vi "Asylum_Driver_InitializeLithographyObject.vi"(6 "Z Setpoint":dbl format="%#_13g", 8 "error in (no error)":errorcluster, 9 "Offsets":cluster{"X":dbl, "Y":dbl}, 10 "Pattern Data":T2={"Name"="", "Litho"=[], "Set Resistance"=enum."1G ohm"}, 11 "Application":refnum<k7>) -> (0 "error out":errorcluster, 3 "Application":refnum<k7>)   [LabVIEW 2020]
uses:
  <userlib>/LevyLab/Relay Box/Type_defs/Resistor--enum.ctl
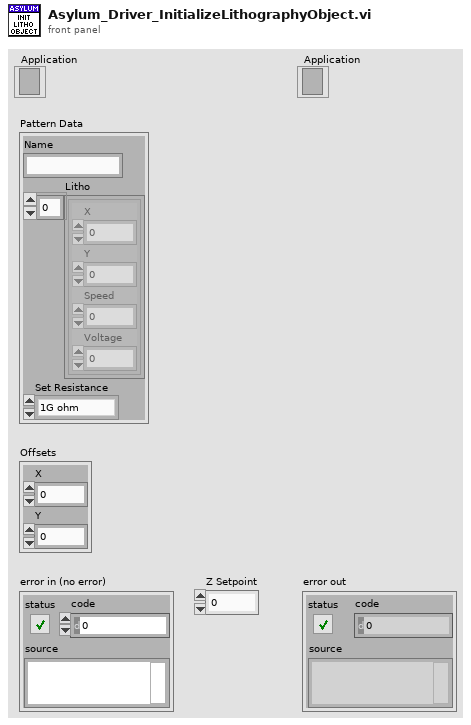
[diagram p1: front panel]
types:
  T1 = typedef "Resistor--enum.ctl" = enum16{"open", "discharge tip", "0 ohms", "100k ohm", "10M ohm", "1G ohm"}
  T2 = cluster{"Name":string, "Litho":cluster{"X":dbl, "Y":dbl, "Speed":dbl, "Voltage":dbl}[], "Set Resistance":T1}
  T3 = cluster{"X":dbl, "Y":dbl, "Speed":dbl, "Voltage":dbl}[]
  T4 = cluster{"X":dbl, "Y":dbl, "Speed":dbl, "Voltage":dbl}
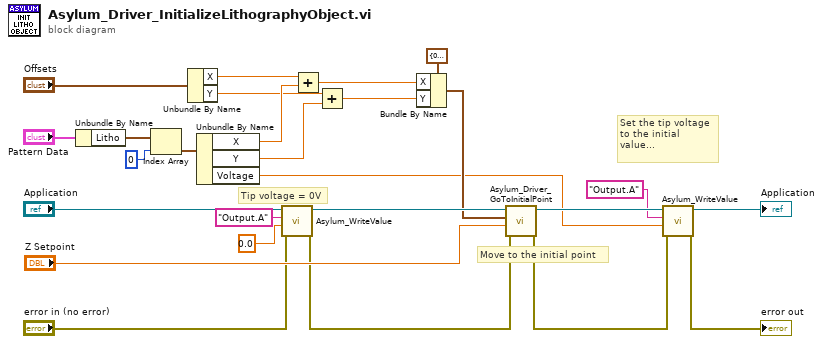
[diagram p0: block diagram]
diagram:
  # "Move to the initial point"
  # "Set the tip voltage to the initial value..."
  # "Tip voltage = 0V"
  n1 = Unbundle By Name("Pattern Data") -> ("Litho"=w20:T3)
  n2 = Index Array(array=w20, index=0) -> (element=w18:T4)
  n3 = Unbundle By Name("Offsets") -> ("X"=w22:dbl, "Y"=w21:dbl)
  n4 = Unbundle By Name(w18) -> ("X"=w24:dbl, "Y"=w23:dbl, "Voltage"=w1:dbl)
  n5 = call <vilib>:"Asylum_WriteValue.vi"("error in (no error)"="error in (no error)", "value"=0.0, "parameterName"="Output.A", "Application"="Application") -> ("error out"=w7:errorcluster, "Application"=w11:refnum<k7>)  [unwired: 6 in]
  n6 = Add(x=w22, y=w24) -> (x+y=w14:dbl)
  n7 = Add(x=w21, y=w23) -> (x+y=w13:dbl)
  n8 = Bundle By Name(cluster=cluster{"X":dbl, "Y":dbl, "Speed":dbl} {"X"=0.0, "Y"=0.0, "Speed"=0.0} ("Coordinate"), "X"=w14, "Y"=w13) -> (w9:cluster{"X":dbl, "Y":dbl, "Speed":dbl})
  n9 = call "Asylum_Driver_GoToInitialPoint.vi"("error in (no error)"=w7, "Z Setpoint"="Z Setpoint", "Coordinate"=w9, "Application"=w11) -> ("error out"=w4:errorcluster, "Application"=w6:refnum<k7>)  [unwired: 6 in]
  n10 = call <vilib>:"Asylum_WriteValue.vi"("error in (no error)"=w4, "value"=w1, "parameterName"="Output.A", "Application"=w6) -> ("error out"=→"error out":errorcluster, "Application"=→"Application":refnum<k7>)  [unwired: 6 in]
